vi "powerVsModFreq_withScopeTraces.vi"() -> ()   [LabVIEW 2016]
uses:
  <vilib>/Utility/file.llb/Write Delimited Spreadsheet (DBL).vi
panel:
  out "time/measurement setting (ms)":u32[](array[numeric])
  in  "num. measmts./setting":i32=10
  out "counter":i32
  out "Current freq.":dbl
  in  "file to save power meter readings to:":path
  in  "Freq step":i32=100000 format="%.2e"
  in  "End freq":dbl=20000000.0 format="%0.2e"
  in  "Start freq":dbl=100000.0 format="%0.2e"
  in  "Shuffle?":bool
  out "IDN String":string
  out "Sensor SN":string
  out "Sensor Name":string
  out "Sensor Flags":bool[](array[boolean])
  out "Readout string":string
  out "Readout value":dbl format="%^#_9e"
  in  "Timeout [ms]":i32=1000
  out "New":bool
  in  "Readout Config":string(combo)="POW"
  in  "Averaging Rate":i32=300
  out "Error log":string
  in  "Enum":enum16{"Triangle", "Sine"}(ring)
  in  "VISA resource name":refnum<visa-resource-name>="GPIB0::4::INSTR"
  in  "Serial Configuration":T1={"Baud Rate"=9600, "Parity"=0, "Data Bits"=8, "Flow Control"=4} {"Flow Control" items=["None", "XON/XOFF", "RTS/CTS", "XON/XOFF & RTS/CTS", "DTR/DSR", "XON/XOFF & DTR/DSR"]; "Data Bits" items=["7"=7, "8"=8]; "Parity" items=["None", "Odd", "Even", "Mark", "Space"]; "Baud Rate" items=["300"=300, "600"=600, "1200"=1200, "2400"=2400, "4800"=4800, "9600"=9600, "19200"=19200]}
  # "(last reading at the bottom of the list)"
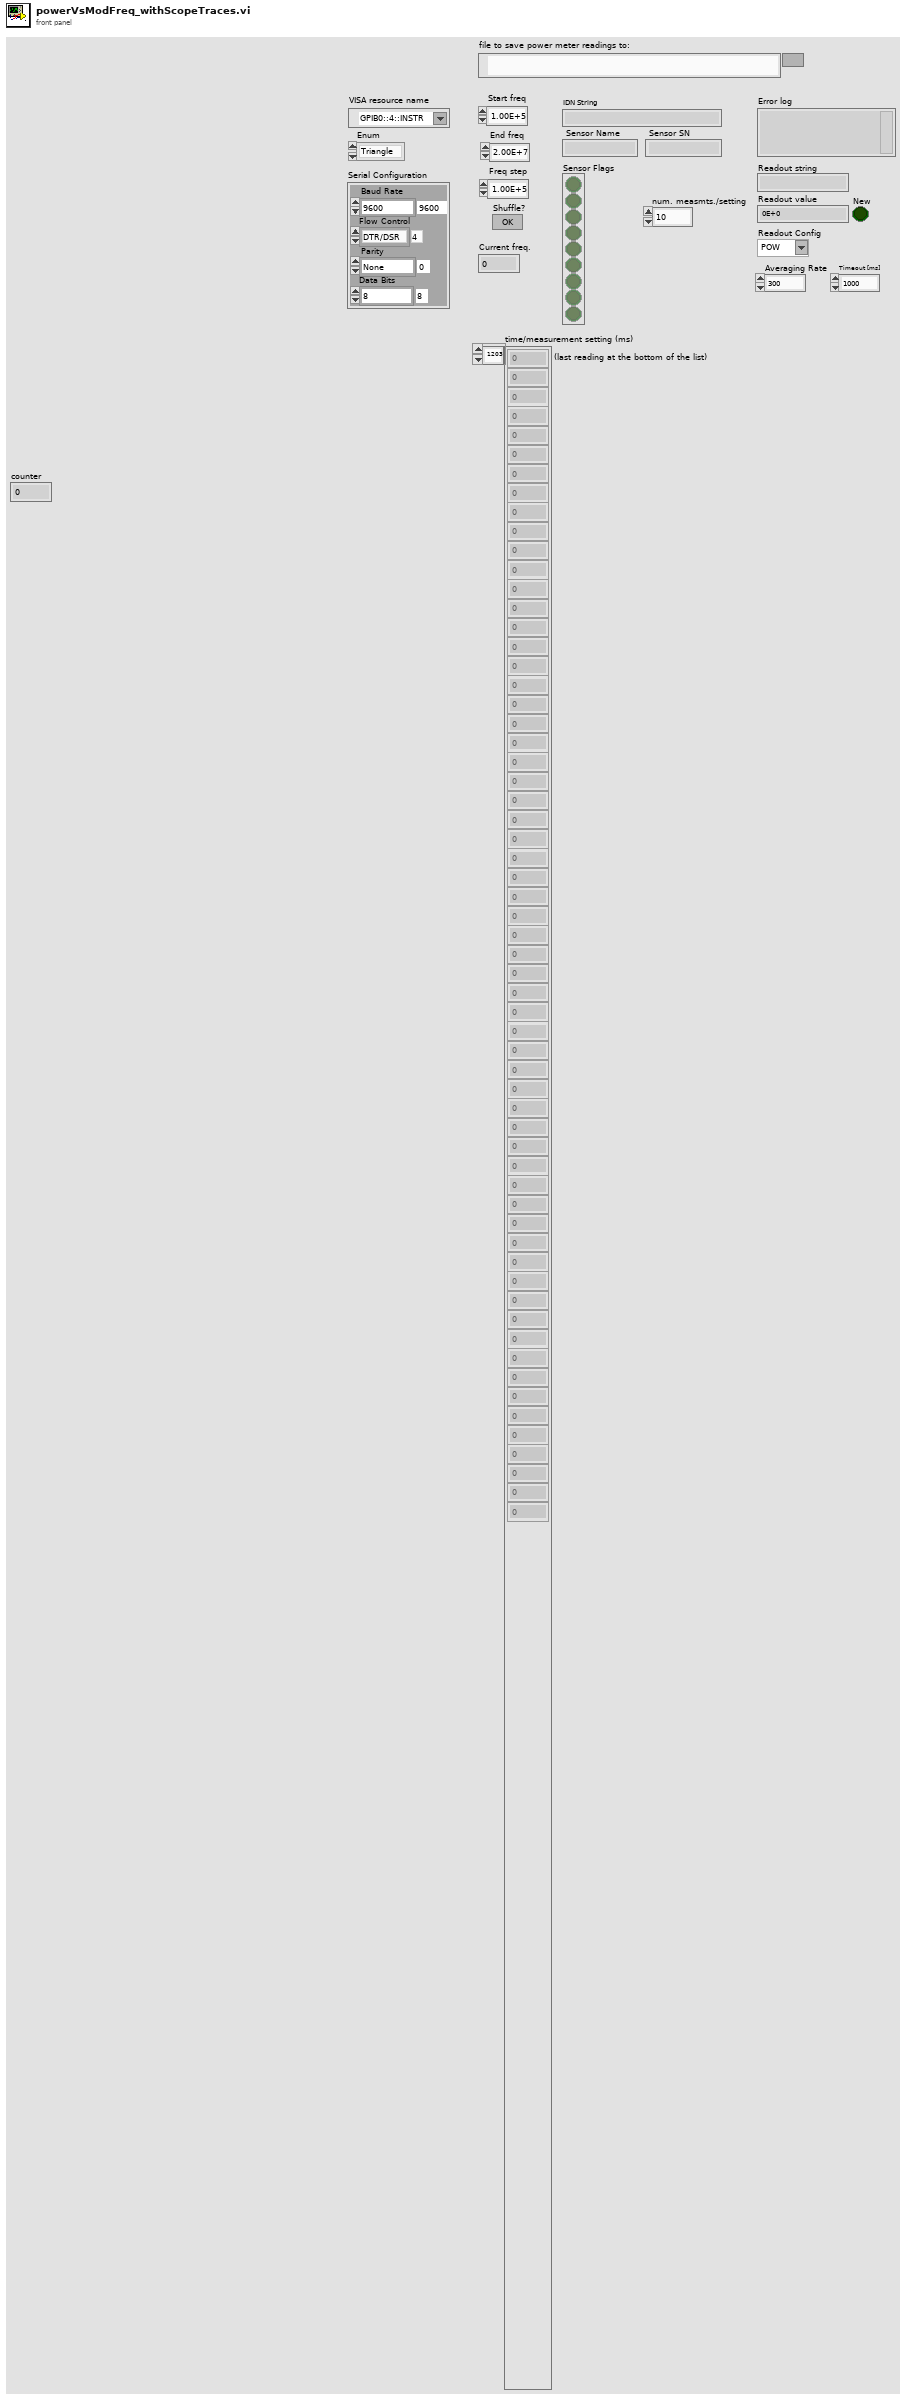
[diagram p1: front panel]
types:
  T1 = cluster{"Baud Rate":u32, "Parity":u16, "Data Bits":u16, "Flow Control":u16}
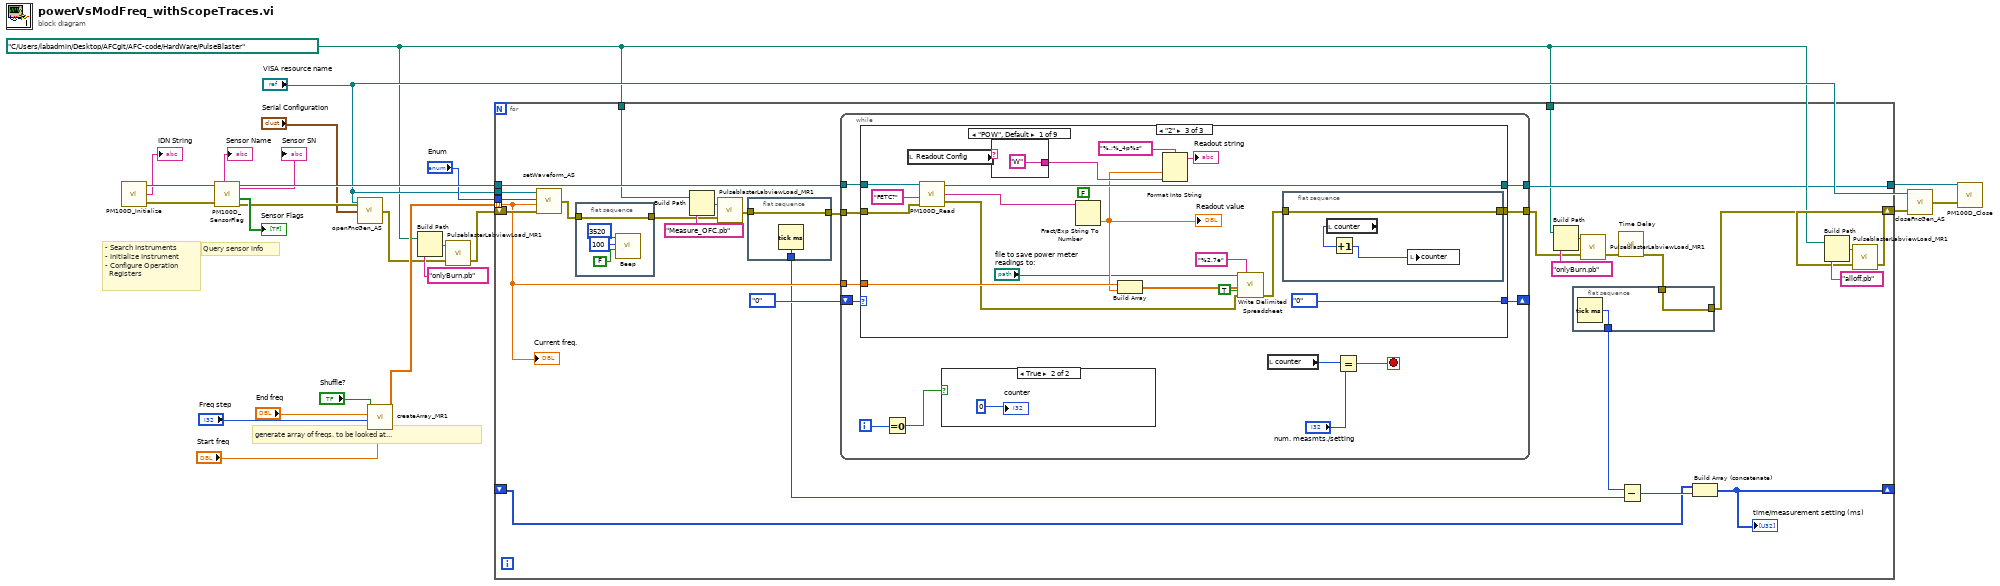
[diagram p0: block diagram]
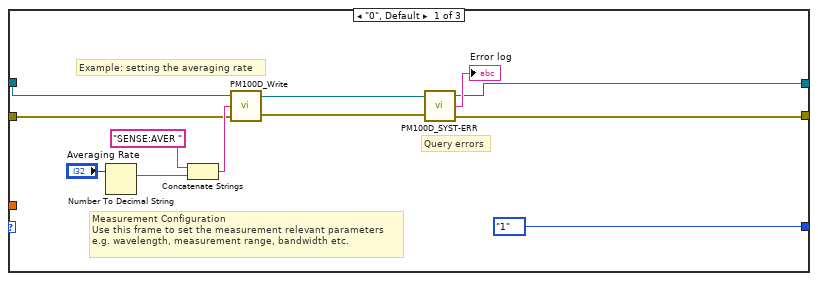
[diagram p3: hidden frame]
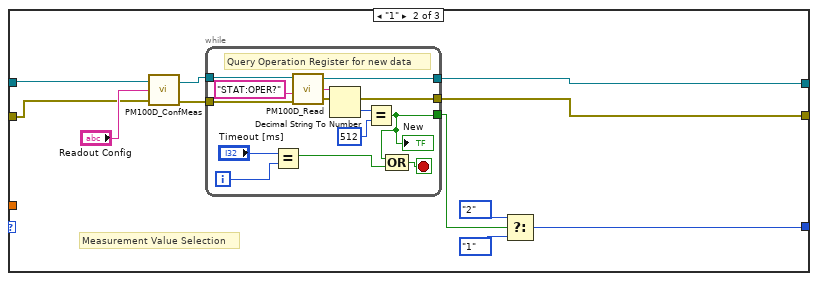
[diagram p4: hidden frame]
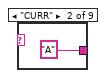
[diagram p5: hidden frame]
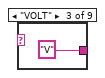
[diagram p6: hidden frame]
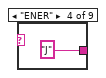
[diagram p7: hidden frame]
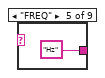
[diagram p8: hidden frame]
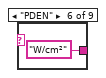
[diagram p9: hidden frame]
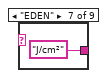
[diagram p10: hidden frame]
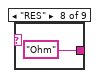
[diagram p11: hidden frame]
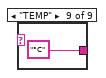
[diagram p12: hidden frame]
diagram:
  w1 = path "C:/Users/labadmin/Desktop/AFCgit/AFC-code/HardWare/PulseBlaster" ("base path")
  # "generate array of freqs. to be looked at..."
  # "- Search Instruments\n- Initialize Instrument\n- Configure Operation\n  Registers"
  # "Query sensor info"
  n1 = call "PM100D_Initialize.vi"() -> ("error out"=w26:errorcluster, "Instrument"=→"IDN String":string, "VISA out"=w27:refnum<visa-resource-name>)  [unwired: 2 in, 1 out]
  n2 = call "PM100D_SensorFlag.vi"("error in (no error)"=w26, "VISA in"=w27) -> ("error out"=w20:errorcluster, "flags"=→"Sensor Flags":bool[], "VISA out"=w25:refnum<visa-resource-name>, "sn"=→"Sensor SN":string, "name"=→"Sensor Name":string)  [unwired: 2 in, 3 out]
  n3 = call "openFncGen_AS.vi"("error in (no error)"=w20, "Serial Configuration"="Serial Configuration", "VISA resource name"="VISA resource name") -> ("error out"=w7:errorcluster)
  n4 = call "createArray_MR1.vi"("Start freq"="Start freq", "Freq step"="Freq step", "End freq"="End freq", "Shuffle?"="Shuffle?") -> ("Riffled {X}"=w14:dbl[])  [unwired: 7 in]
  n5 = Build Path(base path=w1, name or relative path="onlyBurn.pb") -> (appended path=w9:path)
  n6 = call "PulseblasterLabviewLoad_MR1.vi"("error in (no error)"=w7, "Input file"=w9) -> ("error out"=w6:errorcluster)  [unwired: 1 out]
  n7 = for {
    tunnel: w25 -> [w46]
    tunnel: w14 -> [w49] mode=indexing
    tunnel: "VISA resource name" -> [w51]
    tunnel: "Enum" -> [w50]
    tunnel: [w44] -> w10
    shift-right: [w31] -> w3
    shift-left: w6 -> [w52]
    tunnel: w1 -> [w45]
    tunnel: w1 -> [w36]
    shift-right: [w28] -> _
    shift-left: _ -> [w29]
    n8 = call "setWaveform_AS.vi"("error in (no error)"=w52, "Frequency (1000 Hz)"=w49, "Enum"=w50, "VISA resource name"=w51) -> ("error out"=w43:errorcluster)
    n9 = flat-sequence {
      tunnel: w43 -> [w58]
      tunnel: [w58] -> w42
      frame #0 {
        n10 = call <vilib>:"Beep.vi"("use system alert? (T)"=FALSE, "duration (msec)"=u32 100, "frequency (Hz)"=u32 3520) -> ()  [unwired: 9 in]
      }
    }
    n11 = Build Path(base path=w45, name or relative path="Measure_OFC.pb") -> (appended path=w48:path)
    n12 = call "PulseblasterLabviewLoad_MR1.vi"("error in (no error)"=w42, "Input file"=w48) -> ("error out"=w41:errorcluster)  [unwired: 1 out]
    n13 = flat-sequence {
      tunnel: w41 -> [w57]
      tunnel: [w57] -> w40
      tunnel: [w56] -> w39
      frame #0 {
        n14 = Tick Count (ms)() -> (millisecond timer value=w56:u32)
      }
    }
    n15 = while {
      tunnel: w46 -> [w63]
      shift-right: [w72] -> _
      shift-left: enum16{"0", "1", "2"}."0" -> [w73]
      tunnel: [w71] -> w44
      tunnel: [w70] -> w34
      tunnel: w49 -> [w69]
      tunnel: w40 -> [w62]
      i -> [w65]
      stop <- w68 stop-if-true
      n16 = case shown="\"2\"" w73 {
        tunnel: w63 -> [w83 w97 w128]
        tunnel: [enum16{"0", "1", "2"}."1" w92 enum16{"0", "1", "2"}."0"] -> w72
        tunnel: [w77 w94 w127] -> w71
        tunnel: [w76 w93 w112] -> w70
        tunnel: w69 -> [_ _ w118]
        tunnel: w62 -> [w75 w87 w111]
        frame "0", Default {
          # "Query errors"
          # "Example: setting the averaging rate"
          # "Measurement Configuration\nUse this frame to set the measurement relevant parameters\ne.g. wavelength, measurement range, bandwidth etc."
          n17 = Number To Decimal String(number="Averaging Rate") -> (decimal integer string=w85:string)  [unwired: 1 in]
          n18 = Concatenate Strings("SENSE:AVER " ("string"), w85) -> (w82:string)
          n19 = call "PM100D_Write.vi"("error in (no error)"=w75, "Command"=w82, "VISA in"=w83) -> ("error out"=w79:errorcluster, "VISA out"=w81:refnum<visa-resource-name>)
          n20 = call "PM100D_SYST-ERR.vi"("error out 2"=w79, "VISA In"=w81) -> ("error out"=w76:errorcluster, "Error"=→"Error log":string, "VISA Out"=w77:refnum<visa-resource-name>)  [unwired: 1 in]
        }
        frame "1" {
          # "Measurement Value Selection"
          n21 = call "PM100D_ConfMeas.vi"("error in"=w87, "Conf:"="Readout Config", "VISA In"=w97) -> ("error out"=w95:errorcluster, "dup VISA session"=w96:refnum<visa-resource-name>)
          n22 = while {
            tunnel: w96 -> [w106]
            tunnel: w95 -> [w105]
            tunnel: [w104] -> w94
            tunnel: [w103] -> w93
            tunnel: [w98] -> w89
            i -> [w100]
            stop <- w102 stop-if-true
            # "Query Operation Register for new data"
            n23 = Equal?(x="Timeout [ms]", y=w100) -> (x = y?=w99:bool)
            n24 = call "PM100D_Read.vi"("error in (no error)"=w105, "Command"="STAT:OPER?", "VISA in"=w106) -> ("error out"=w103:errorcluster, "ReadValue"=w109:string, "VISA out"=w104:refnum<visa-resource-name>)  [unwired: 1 in]
            n25 = Decimal String To Number(string=w109) -> (number=w108:i32)  [unwired: 2 in, 1 out]
            n26 = Equal?(x=w108, y=512) -> (x = y?=w98:bool)
            "New" <- w98
            n27 = Compound Arithmetic op=OR(w98, w99) -> (w102:bool)
          }
          n28 = Select(t=enum16{"0", "1", "2"}."2", s=w89, f=enum16{"0", "1", "2"}."1") -> (s? t:f=w92:enum16{"0", "1", "2"})
        }
        frame "2" {
          n29 = local read "Readout Config"() -> (w126:string)
          n30 = call "PM100D_Read.vi"("error in (no error)"=w111, "Command"="FETC?", "VISA in"=w128) -> ("error out"=w114:errorcluster, "ReadValue"=w125:string, "VISA out"=w127:refnum<visa-resource-name>)  [unwired: 1 in]
          n31 = case shown="\"POW\", Default" w126 {
            tunnel: ["W" "A" "V" "J" "Hz" "W/cm²" "J/cm²" "Ohm" "°C"] -> w122
            frame "POW", Default {
            }
            frame "CURR" {
            }
            frame "VOLT" {
            }
            frame "ENER" {
            }
            frame "FREQ" {
            }
            frame "PDEN" {
            }
            frame "EDEN" {
            }
            frame "RES" {
            }
            frame "TEMP" {
            }
          }
          n32 = Fract/Exp String To Number(use system decimal point (T)=FALSE, string=w125) -> (number=w117:dbl)  [unwired: 2 in, 1 out]
          "Readout value" <- w117
          n33 = Build Array(w118, w117) -> (w116:dbl[])
          n34 = Format Into String(format string="%.;%_4p%s", w117, w122) -> (resulting string=→"Readout string":string)  [unwired: 2 in, 1 out]
          n35 = call-poly <vilib>:"Write Delimited Spreadsheet.vi"("file path (dialog if empty)"="file to save power meter readings to:", "format (%.3f)"="%2.7e", "1D data"=w116, "append to file? (new file:F)"=TRUE, "error in (no error)"=w114) -> ("error out"=w113:errorcluster)  [unwired: 9 in, 1 out]
          n36 = flat-sequence {
            tunnel: w113 -> [w133]
            tunnel: [w133] -> w112
            frame #0 {
              n37 = local read "counter"() -> (w132:i32)
              n38 = Increment(x=w132) -> (x+1=w131:i32)
              n39 = local write "counter"(w131) -> ()
            }
          }
        }
      }
      n40 = Equal To 0?(x=w65) -> (x = 0?=w66:bool)
      n41 = case shown="True" w66 {
        frame False {
        }
        frame True {
          "counter" <- 0 ("counter")
        }
      }
      n42 = local read "counter"() -> (w64:i32)
      n43 = Equal?(x=w64, y="num. measmts./setting") -> (x = y?=w68:bool)
    }
    n44 = Build Path(base path=w36, name or relative path="onlyBurn.pb") -> (appended path=w38:path)
    n45 = flat-sequence {
      tunnel: [w55] -> w32
      tunnel: w33 -> [w54]
      tunnel: [w54] -> w31
      frame #0 {
        n46 = Tick Count (ms)() -> (millisecond timer value=w55:u32)
      }
    }
    n47 = call "PulseblasterLabviewLoad_MR1.vi"("error in (no error)"=w34, "Input file"=w38) -> ("error out"=w35:errorcluster)  [unwired: 1 out]
    n48 = call "Time Delay"("error in (no error)"=w35) -> ("error out"=w33:errorcluster)  [unwired: 10 in]
    n49 = Subtract(x=w32, y=w39) -> (x-y=w30:u32)
    n50 = Build Array (concatenate)(w29, w30) -> (w28:u32[])
    "time/measurement setting (ms)" <- w28
    "Current freq." <- w49
  }
  n51 = Build Path(base path=w1, name or relative path="alloff.pb") -> (appended path=w5:path)
  n52 = call "PulseblasterLabviewLoad_MR1.vi"("error in (no error)"=w3, "Input file"=w5) -> ("error out"=w2:errorcluster)  [unwired: 1 out]
  n53 = call "closeFncGen_AS.vi"("error in (no error)"=w2, "VISA resource name"="VISA resource name") -> ("error out"=w11:errorcluster)  [unwired: 1 in]
  n54 = call "PM100D_Close.vi"("error in (no error)"=w11, "VISA resource name"=w10) -> ()  [unwired: 2 in]
